vi "AprilTag Target Package Code 2.vi"() -> ()   [LabVIEW 2023]
uses:
  Camera Info.ctl
  State Machine/AprialTag Main Cluster.ctl
  State Machine/AprialTag States.ctl
  <vilib>/vision/Image Controls.llb/IMAQ Image.ctl
  Steam Type.ctl
  Camera Set Up/Event Setup Types.ctl
  <vilib>/Utility/config.llb/Read Key (String).vi
  <vilib>/Utility/config.llb/Write Key (String).vi
  <vilib>/Utility/config.llb/NI_LVConfig.lvlib
panel:
  in  "Main":enum32{"Page 1", "Page 2"}(tab)
  out "Target Pitch":dbl[](array[numeric]) caption="Tag Pitch (deg)" format="%.1f"
  out "Target Roll":dbl[](array[numeric]) caption="Tag Yaw (deg)" format="%.1f"
  out "Tag ID":dbl[](array[numeric]) caption="Tag Number"
  out "Image":T1(plugin-control)
  in  "Camera Name":string="cam0"
  in  "Settings":bool
  in  "Save":bool
  in  "Tools":bool
  out "AprilTag Fps":dbl format="%#.0f"
  out "Distance":dbl[](array[numeric]) caption="Tag Distance (in)" format="%.1f"
  out "Angle":dbl[](array[numeric]) caption="Center Angle (deg)" format="%.1f"
  in  "Home":bool
  in  "FOV":dbl=68.5
  in  "Robot Calibration Cluster":T2={"Camera Height on robot (in)"=9.5, "Camera Angle on the robot (deg)"=2.5, "Camera FOV Top to Bottom View Angle (deg)"=26.5, "Target size (in)"=6.5, "Distance to front of bumper (in)"=9.75, "Focal Length (mm)"=10.0, "Yaw Slope"=0.0} {"Focal Length (mm)" format="%#_13g"; "Distance to front of bumper (in)" format="%#_13g"; "Target size (in)" format="%#_13g"; "Camera FOV Top to Bottom View Angle (deg)" format="%#_13g"; "Camera Angle on the robot (deg)" format="%#_13g"; "Camera Height on robot (in)" format="%#_13g"}
  # "Edit the camera name to the camera that you are going to use for this target package"
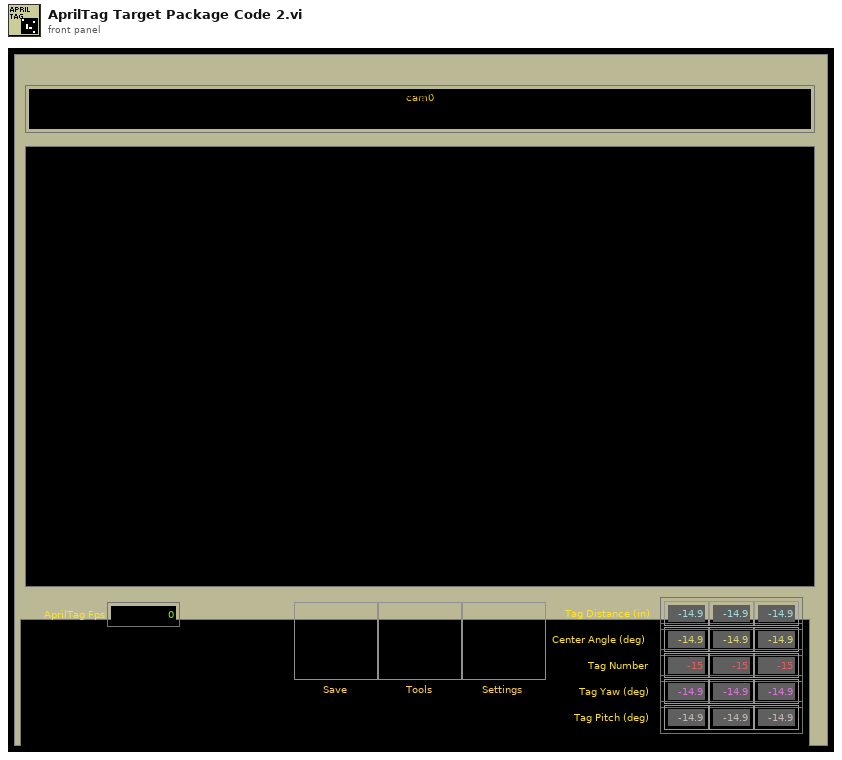
[diagram p1: front panel]
types:
  T1 = typedef "IMAQ Image.ctl" = refnum<image>
  T2 = typedef "Camera Info.ctl" = cluster{"Camera Height on robot (in)":dbl, "Camera Angle on the robot (deg)":dbl, "Camera FOV Top to Bottom View Angle (deg)":dbl, "Target size (in)":dbl, "Distance to front of bumper (in)":dbl, "Focal Length (mm)":dbl, "Yaw Slope":dbl}
  T3 = typedef "AprialTag States.ctl" = enum16{"Message Dispatcher", "INI", "Open", "Save", "Exit"}
  T4 = typedef "AprialTag Main Cluster.ctl" = cluster{"AprilTage FIFO":T3[], "Camera Name":string, "AprilTag path":path, "Control Ref's":refnum<vi>[], "Calibration Mask":T1, "Main Image":T1, "Timeout":i32, "EDIT Settings":bool, "Calibration path":path, "Camera Number":dbl}
  T5 = typedef "Steam Type.ctl" = enum8{"Unknown", "Apriltag", "Algae", "Coral"}
  T6 = typedef "Event Setup Types.ctl" = enum16{"Default", "Camera Loop Started", "Close Settings", "GreyScale", "Open Front Panel", "Save Data", "Exit"}
  T7 = cluster{"tag ID":i32, "Center":cluster{"X":dbl, "Y":dbl}, "homography matrix":dbl[], "decision margin":dbl, "Hamming Dist":i32, "corner points":cluster{"X":dbl, "Y":dbl}[], "Tag Family":string}[]
  T8 = typedef "AprilTag Target Fields.ctl" = cluster{"diameter points":cluster{"first point":cluster{"x":dbl, "y":dbl}, "projected point":cluster{"x":dbl, "y":dbl}}, "normalized center":cluster{"x":dbl, "y":dbl}, "Overall Score":dbl, "Distance (ft)":dbl, "Offset Angle":dbl, "Tag corner points":cluster{"X":dbl, "Y":dbl}[], "Tag Center":cluster{"X":dbl, "Y":dbl}, "Tag Yaw":dbl, "Tag Pitch":dbl, "AprilTag Number":i32}
  T9 = typedef "Image Type" = u32
  T10 = typedef "NI_LVConfig.lvlib/Config Data RefNum.ctl" = refnum<k1>
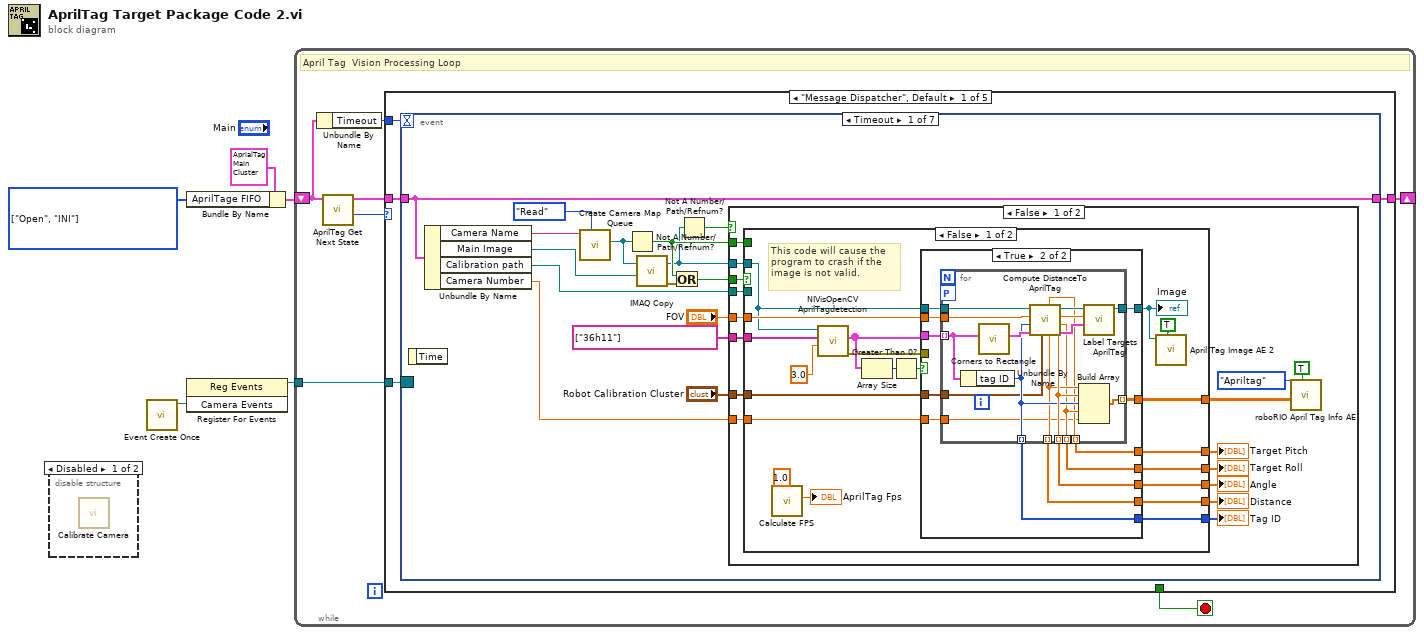
[diagram p0: block diagram]
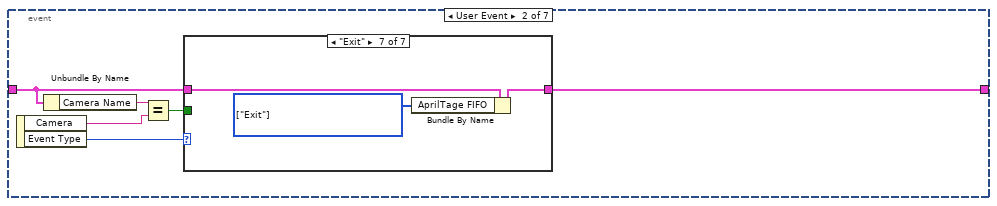
[diagram p6: hidden frame]
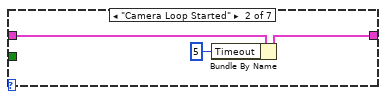
[diagram p8: hidden frame]
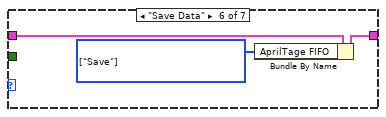
[diagram p12: hidden frame]
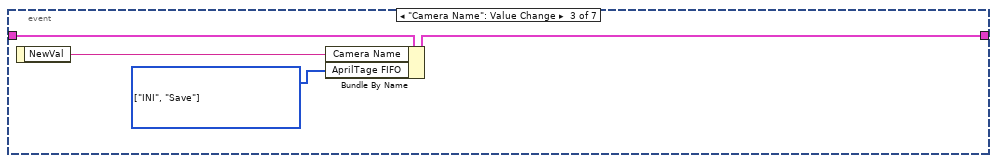
[diagram p13: hidden frame]
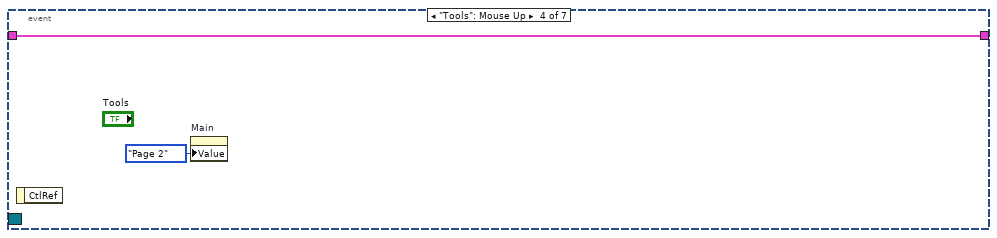
[diagram p14: hidden frame]
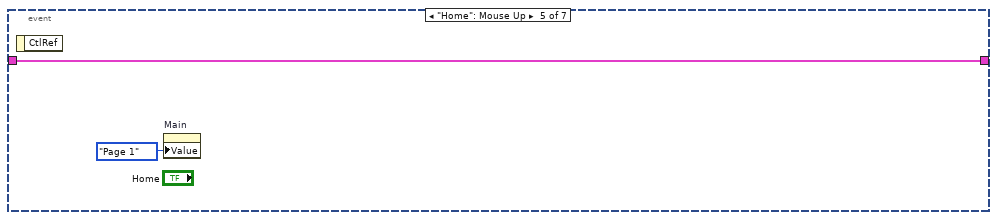
[diagram p15: hidden frame]
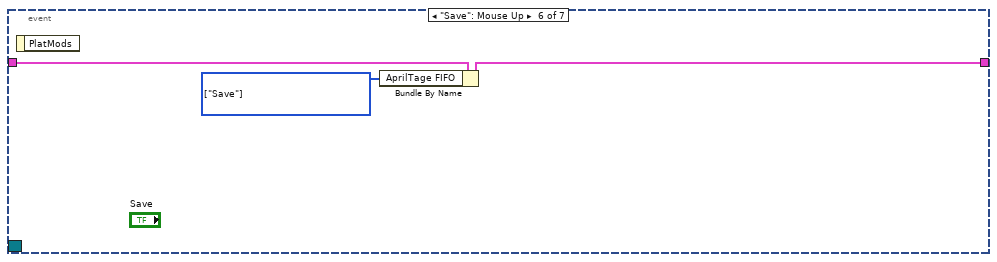
[diagram p16: hidden frame]
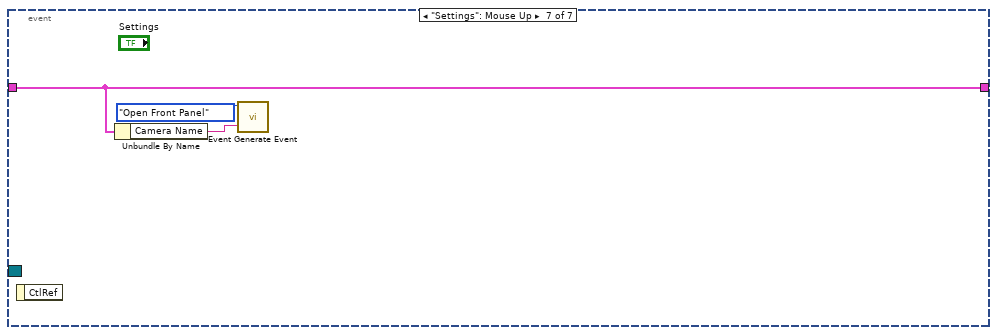
[diagram p17: hidden frame]
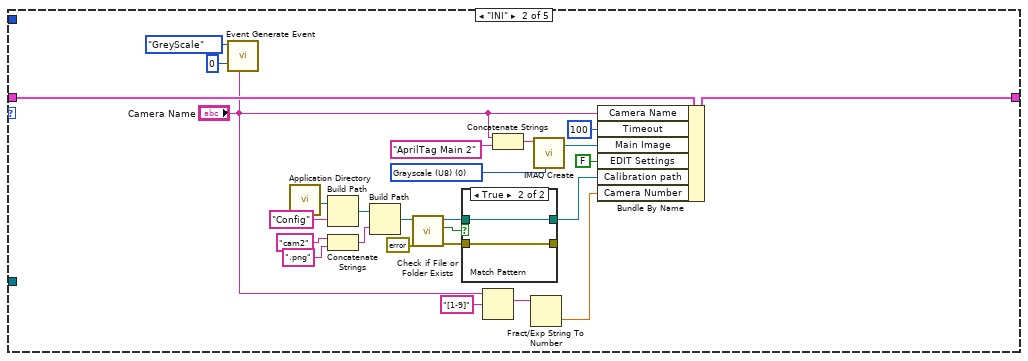
[diagram p18: hidden frame]
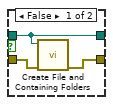
[diagram p19: hidden frame]
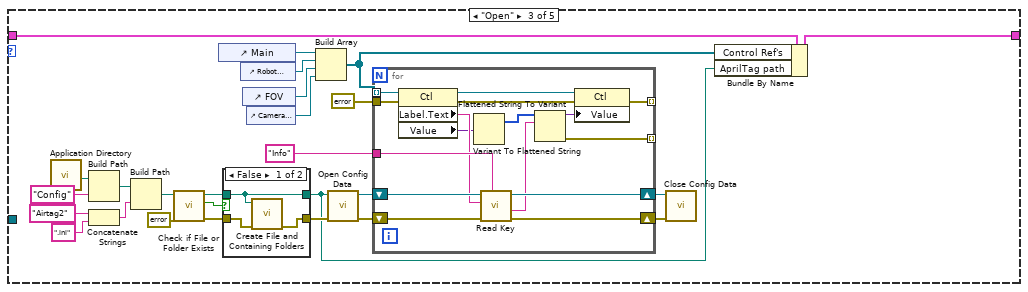
[diagram p20: hidden frame]
diagram:
  w1 = T3[] [enum."Open", enum."INI"] items=["Message Dispatcher", "INI", "Open", "Save", "Exit"] ("AprilTage FIFO")
  n1 = disable-structure shown="Disabled" {
    frame Disabled {
      n2 = call "Calibrate Camera.vi"() -> ()  [unwired: 13 in, 3 out]
    }
    frame Enabled {
    }
  }
  n3 = call "Event Create Once.vi"() -> ("Camera Events"=w5:refnum<user-event>)  [unwired: 10 in, 1 out]
  n4 = Bundle By Name(cluster=T4 {"AprilTage FIFO"=[], "Camera Name"="", "AprilTag path"=path "", "Control Ref's"=[], "Calibration Mask"=refnum, "Main Image"=refnum, "Timeout"=5, "EDIT Settings"=FALSE, "Calibration path"=path "", "Camera Number"=0.0} ("AprilTag Main Cluster out"), "AprilTage FIFO"=w1) -> (w2:T4)
  n5 = register-events(w5) -> (reference out=w4:refnum<event-registration>)  [unwired: 2 in, 1 out]
  n6 = while {
    tunnel: w4 -> [w12]
    shift-right: [w8] -> _
    shift-left: w2 -> [w6]
    stop <- w11 stop-if-true
    # "April Tag  Vision Processing Loop"
    n7 = Unbundle By Name(w6) -> ("Timeout"=w7:i32)
    n8 = call "AprilTag Get Next State.vi"("AprilTag Main Cluster in"=w6) -> ("Next State"=w9:T3, "AprilTag Main Cluster out"=w10:T4)  [unwired: 9 in]
    n9 = case shown="\"Message Dispatcher\", Default" w9 {
      tunnel: w12 -> [w16 _ _ _ _]
      tunnel: [_ _ _ _ TRUE] -> w11
      tunnel: w10 -> [w14 w154 w171 w210 w227]
      tunnel: [w15 w153 w169 w210 w227] -> w8
      tunnel: w7 -> [w13 _ _ _ _]
      frame "Message Dispatcher", Default {
        n10 = event shown="[0] Timeout" {
          selector: w16 -> [_ _ _ _ _ _ _]
          dyn-events: _ -> [_ _ _ _ _ _ _]
          timeout: w13 -> [_ _ _ _ _ _ _]
          tunnel: w14 -> [w31 w99 w118 w119 w121 w125 w127]
          tunnel: [w31 w101 w117 w119 w121 w124 w127] -> w15
          event Timeout {
            n11 = event-data() -> ()  [unwired: 1 in, 1 out]
            n12 = Unbundle By Name(w31) -> ("Camera Name"=w24:string, "Main Image"=w20:T1, "Calibration path"=w30:path, "Camera Number"=w17:dbl)
            n13 = call "Create Camera Map Queue.vi"("Action"=enum16{"Read", "Write"}."Read", "Camera"=w24) -> ("Image out"=w23:T1)  [unwired: 8 in, 1 out]
            n14 = Not A Number/Path/Refnum?(number/path/refnum=w23) -> (NaN/Path/Refnum?=w26:bool)
            n15 = call "IMAQ Copy"("Image Dst"=w20, "Image Src"=w23) -> ("error out"=w21:errorcluster, "Image Dst Out"=w19:T1)  [unwired: 4 in]
            n16 = Or(x=w26, y=w21) -> (x .or. y?=w22:bool)
            n17 = Not A Number/Path/Refnum?(number/path/refnum=w19) -> (NaN/Path/Refnum?=w18:bool)
            n18 = case shown="False" w18 {
              tunnel: w30 -> [w44 _]
              tunnel: string[] ["36h11"] ("Tag Familys") -> [w43 _]
              tunnel: "FOV" -> [w42 _]
              tunnel: "Robot Calibration Cluster" -> [w41 _]
              tunnel: w26 -> [w40 _]
              tunnel: w22 -> [w34 _]
              tunnel: w19 -> [w33 _]
              tunnel: w17 -> [w32 _]
              frame False {
                n19 = case shown="False" w34 {
                  tunnel: w43 -> [w67 _]
                  tunnel: w42 -> [w66 _]
                  tunnel: w41 -> [w65 _]
                  tunnel: [w56 _] -> w46
                  tunnel: w40 -> [_ _]
                  tunnel: w44 -> [_ _]
                  tunnel: [w55 _] -> w39
                  tunnel: [w54 _] -> w38
                  tunnel: [w53 _] -> w37
                  tunnel: [w52 _] -> w36
                  tunnel: [w51 _] -> w35
                  tunnel: w33 -> [w49 _]
                  tunnel: w32 -> [w48 _]
                  frame False {
                    # "This code will cause the program to crash if the image is not valid."
                    n20 = call "Calculate FPS.vi"("Frames Processed"=1.0) -> ("Fps"=→"AprilTag Fps":dbl)  [unwired: 10 in]
                    n21 = call "NIVisOpenCV AprilTagdetection.vi"("decimate"=3.0, "Tag Familys"=w67, "Image Src"=w49) -> ("error out"=w61:errorcluster, "Detected Tags"=w64:T7)  [unwired: 5 in, 2 out]
                    n22 = Array Size(array=w64) -> (size(s)=w63:i32)
                    n23 = Greater Than 0?(x=w63) -> (x > 0?=w62:bool)
                    n24 = case shown="True" w62 {
                      tunnel: w49 -> [w68 w80]
                      tunnel: w64 -> [_ w79]
                      tunnel: [w68 w78] -> w60
                      tunnel: w61 -> [_ _]
                      tunnel: w66 -> [_ w77]
                      tunnel: w65 -> [_ w76]
                      tunnel: [_ w75] -> w56
                      tunnel: [_ w74] -> w55
                      tunnel: [_ w73] -> w54
                      tunnel: [_ w72] -> w53
                      tunnel: [_ w71] -> w52
                      tunnel: [_ w70] -> w51
                      tunnel: w48 -> [_ w69]
                      frame False {
                      }
                      frame True {
                        n25 = for {
                          tunnel: w79 -> [w93] mode=indexing
                          tunnel: w80 -> [w94]
                          tunnel: [w95] -> w78
                          tunnel: [w87] -> w72 mode=indexing
                          tunnel: [w85] -> w70 mode=indexing
                          tunnel: [w89] -> w71 mode=indexing
                          tunnel: w77 -> [w88]
                          tunnel: w76 -> [w86]
                          tunnel: [w84] -> w73 mode=indexing
                          tunnel: [w83] -> w75 mode=indexing
                          tunnel: [w82] -> w74 mode=indexing
                          workers-P: _ -> [_]
                          tunnel: w69 -> [w81]
                          n26 = Unbundle By Name(w93) -> ("tag ID"=w87:i32)
                          n27 = call "Corners to Rectangle.vi"("tag info"=w93) -> ("output cluster"=w92:T8)  [unwired: 10 in]
                          n28 = call "Compute DistanceTo AprilTag.vi"("Robot Calibration Cluster"=w86, "results"=w92, "AprilTag Number"=w87, "FOV Left to Right (deg)"=w88, "Image Src"=w94) -> ("results out"=w91:T8, "Target Yaw (deg)"=w84:dbl, "Offset Angle"=w89:dbl, "Image Dst Out"=w90:T1, "Distance from target (in)"=w85:dbl, "Target Pitch (deg)"=w82:dbl)  [unwired: 1 in]
                          n29 = Build Array(w85, w89, w87, w84, w81) -> (w83:dbl[])
                          n30 = call "Label Targets AprilTagl.vi"("results"=w91, "Angle"=w89, "Image in"=w90) -> ("Image out"=w95:T1)  [unwired: 8 in]
                        }
                      }
                    }
                    "Image" <- w60
                    n31 = call "April Tag Image AE 2.vi"("Update"=TRUE, "Ball Image in"=w60) -> ()  [unwired: 9 in, 1 out]
                  }
                  frame True {
                  }
                }
                "Distance" <- w35
                "Angle" <- w36
                "Tag ID" <- w37
                "Target Roll" <- w38
                "Target Pitch" <- w39
                n32 = call "roboRIO April Tag Info AE.vi"("Update"=TRUE, "Info in"=w46, "Stream Type"=Steam_Type."Apriltag") -> ()  [unwired: 8 in, 1 out]
              }
              frame True {
              }
            }
          }
          event User Event {
            n33 = event-data() -> ("Camera"=w97:string, "Event Type"=w100:T6)  [unwired: 1 in]
            n34 = Unbundle By Name(w99) -> ("Camera Name"=w98:string)
            n35 = Equal?(x=w98, y=w97) -> (x = y?=w96:bool)
            n36 = case shown="\"Exit\"" w100 {
              tunnel: w99 -> [w102 w105 w106 w107 w108 w111 w114]
              tunnel: [w102 w104 w106 w107 w108 w110 w113] -> w101
              tunnel: w96 -> [_ _ _ _ _ _ _]
              frame "Default" {
              }
              frame "Camera Loop Started" {
                n37 = Bundle By Name(cluster=w105, "Timeout"=5) -> (w104:T4)
              }
              frame "Close Settings" {
              }
              frame "GreyScale" {
              }
              frame "Open Front Panel" {
              }
              frame "Save Data" {
                w109 = T3[] [enum."Save"] items=["Message Dispatcher", "INI", "Open", "Save", "Exit"] ("AprilTage FIFO")
                n38 = Bundle By Name(cluster=w111, "AprilTage FIFO"=w109) -> (w110:T4)
              }
              frame "Exit" {
                w112 = T3[] [enum."Exit"] items=["Message Dispatcher", "INI", "Open", "Save", "Exit"] ("AprilTage FIFO")
                n39 = Bundle By Name(cluster=w114, "AprilTage FIFO"=w112) -> (w113:T4)
              }
            }
          }
          event "Camera Name": Value Change {
            w116 = T3[] [enum."INI", enum."Save"] items=["Message Dispatcher", "INI", "Open", "Save", "Exit"] ("AprilTage FIFO")
            n40 = event-data() -> ("NewVal"=w115:string)  [unwired: 1 in]
            n41 = Bundle By Name(cluster=w118, "Camera Name"=w115, "AprilTage FIFO"=w116) -> (w117:T4)
          }
          event "Tools": Mouse Up {
            n42 = event-data() -> ()  [unwired: 1 in, 1 out]
            n43 = property on="Main" class="TabCtl (strict)"("Value"=enum32{"Page 1", "Page 2"}."Page 2" ("Main")) -> ()  [unwired: 2 in, 2 out]
          }
          event "Home": Mouse Up {
            n44 = event-data() -> ()  [unwired: 1 in, 1 out]
            n45 = property on="Main" class="TabCtl (strict)"("Value"=enum32{"Page 1", "Page 2"}."Page 1" ("Main")) -> ()  [unwired: 2 in, 2 out]
          }
          event "Save": Mouse Up {
            w123 = T3[] [enum."Save"] items=["Message Dispatcher", "INI", "Open", "Save", "Exit"] ("AprilTage FIFO")
            n46 = event-data() -> ()  [unwired: 1 in, 1 out]
            n47 = Bundle By Name(cluster=w125, "AprilTage FIFO"=w123) -> (w124:T4)
          }
          event "Settings": Mouse Up {
            n48 = event-data() -> ()  [unwired: 1 in, 1 out]
            n49 = Unbundle By Name(w127) -> ("Camera Name"=w126:string)
            n50 = call "Event Generate Event.vi"("Camera Name"=w126, "Event Type"=Event_Setup_Types."Open Front Panel") -> ()  [unwired: 10 in]
          }
        }
      }
      frame "INI" {
        w151 = T9 0 items=["Grayscale (U8)", "Grayscale (I16)", "Grayscale (SGL)", "Complex (CSG)", "RGB (U32)", "HSL (U32)", "RGB (U64)", "Grayscale (U16)"] ("Image Type")
        n51 = call "Event Generate Event.vi"("Camera Name"="Camera Name", "Setpoint"=i64 0, "Event Type"=Event_Setup_Types."GreyScale") -> ()  [unwired: 9 in]
        n52 = call <vilib>:"Application Directory.vi"() -> ("Application Directory"=w144:path)
        n53 = Build Path(base path=w144, name or relative path="Config") -> (appended path=w142:path)
        n54 = Concatenate Strings("cam2" ("string"), ".png" ("name or relative path")) -> (w146:string)
        n55 = Build Path(base path=w142, name or relative path=w146) -> (appended path=w141:path)
        n56 = call <vilib>:"Check if File or Folder Exists.vi"("error in (no error)"=errorcluster {"status"=FALSE, "code"=0, "source"=""}, "path"=w141) -> ("error out"=w138:errorcluster, "file or folder exists?"=w139:bool, "dup path"=w140:path)  [unwired: 7 in]
        n57 = case shown="True" w139 {
          tunnel: [w157 w158] -> _
          tunnel: w140 -> [w156 w159]
          tunnel: [w156 w159] -> w135
          tunnel: w138 -> [w155 w158]
          frame False {
            n58 = call <vilib>:"Create File and Containing Folders.vi"("error in (no error)"=w155, "file path"=w156) -> ("error out"=w157:errorcluster)  [unwired: 8 in, 1 out]
          }
          frame True {
          }
        }
        n59 = Match Pattern(string="Camera Name", regular expression="[1-9]") -> (match substring=w131:string)  [unwired: 1 in, 3 out]
        n60 = Concatenate Strings("Camera Name", "AprilTag Main 2" ("string")) -> (w150:string)
        n61 = Fract/Exp String To Number(string=w131) -> (number=w129:dbl)  [unwired: 3 in, 1 out]
        n62 = call "IMAQ Create"("Image Name"=w150, "Image Type"=w151) -> ("New Image"=w148:T1)  [unwired: 2 in, 2 out]
        n63 = Bundle By Name(cluster=w154, "Camera Name"="Camera Name", "Timeout"=100, "Main Image"=w148, "EDIT Settings"=FALSE, "Calibration path"=w135, "Camera Number"=w129) -> (w153:T4)
      }
      frame "Open" {
        n64 = call <vilib>:"Application Directory.vi"() -> ("Application Directory"=w174:path)
        n65 = Build Path(base path=w174, name or relative path="Config") -> (appended path=w172:path)
        n66 = Concatenate Strings("Airtag2" ("string"), ".ini" ("name or relative path")) -> (w185:string)
        n67 = Build Path(base path=w172, name or relative path=w185) -> (appended path=w165:path)
        n68 = call <vilib>:"Check if File or Folder Exists.vi"("error in (no error)"=errorcluster {"status"=FALSE, "code"=0, "source"=""}, "path"=w165) -> ("error out"=w161:errorcluster, "file or folder exists?"=w163:bool, "dup path"=w164:path)  [unwired: 7 in]
        n69 = control-ref of="Main"() -> (w180:refnum<vi>)
        n70 = case shown="False" w163 {
          tunnel: [w188 w189] -> w175
          tunnel: w164 -> [w187 w190]
          tunnel: [w187 w190] -> w162
          tunnel: w161 -> [w186 w189]
          frame False {
            n71 = call <vilib>:"Create File and Containing Folders.vi"("error in (no error)"=w186, "file path"=w187) -> ("error out"=w188:errorcluster)  [unwired: 8 in, 1 out]
          }
          frame True {
          }
        }
        n72 = control-ref of="Robot Calibration Cluster"() -> (w179:refnum<vi>)
        n73 = control-ref of="FOV"() -> (w178:refnum<vi>)
        n74 = control-ref of="Camera Name"() -> (w170:refnum<vi>)
        n75 = Build Array(w180, w179, w178, w170) -> (w168:refnum<vi>[])
        n76 = call <vilib>:"Open Config Data.vi"("error in (no error)"=w175, "configuration file path"=w162) -> ("error out"=w181:errorcluster, "refnum"=w184:T10)  [unwired: 7 in, 1 out]
        n77 = for {
          tunnel: "Info" ("Camera Name") -> [w203]
          tunnel: w168 -> [w201] mode=indexing
          shift-right: [w205] -> w183
          shift-left: w184 -> [w206]
          shift-right: [w204] -> w182
          shift-left: w181 -> [w202]
          tunnel: [w196] -> _ mode=indexing
          tunnel: errorcluster {"status"=FALSE, "code"=0, "source"=""} ("error out") -> [w195]
          tunnel: [w191] -> _ mode=indexing
          n78 = property class="Ctl"(reference=w201, error in=w195) -> (reference out=w199:refnum<vi>, error out=w197:errorcluster, "Label.Text"=w200:string, "Value"=w193:variant)
          n79 = Variant To Flattened String(Variant=w193) -> (1:w192:i16[])  [unwired: 1 out]
          n80 = call-poly <vilib>:"Read Key.vi"("section"=w203, "error in (no error)"=w202, "key"=w200, "refnum"=w206) -> ("error out"=w204:errorcluster, "value"=w198:string, "refnum out"=w205:T10)  [unwired: 4 in, 1 out]
          n81 = Flattened String To Variant(6:w198, 7:w192) -> (0:w191:errorcluster, 3:w194:variant)  [unwired: 1 in]
          n82 = property class="Ctl"(reference=w199, error in=w197, "Value"=w194) -> (error out=w196:errorcluster)  [unwired: 1 out]
        }
        n83 = call <vilib>:"Close Config Data.vi"("error in (no error)"=w182, "refnum"=w183) -> ()  [unwired: 8 in, 2 out]
        n84 = Bundle By Name(cluster=w171, "Control Ref's"=w168, "AprilTag path"=w162) -> (w169:T4)
      }
      frame "Save" {
        n85 = Unbundle By Name(w210) -> ("Control Ref's"=w208:refnum<vi>[], "AprilTag path"=w209:path)
        n86 = call <vilib>:"Open Config Data.vi"("configuration file path"=w209) -> ("error out"=w211:errorcluster, "refnum"=w214:T10)  [unwired: 8 in, 1 out]
        n87 = for {
          tunnel: "Info" ("Camera Name") -> [w220]
          shift-right: [w223] -> w213
          shift-left: w214 -> [w224]
          shift-right: [w222] -> w212
          shift-left: w211 -> [w221]
          tunnel: w208 -> [w215] mode=indexing
          n88 = property class="Ctl"(reference=w215, error in=w221) -> (error out=w217:errorcluster, "Label.Text"=w219:string, "Value"=w218:variant)  [unwired: 1 out]
          n89 = Variant To Flattened String(Variant=w218) -> (data string=w216:string)  [unwired: 1 out]
          n90 = call-poly <vilib>:"Write Key.vi"("section"=w220, "error in (no error)"=w217, "value"=w216, "key"=w219, "refnum"=w224) -> ("error out"=w222:errorcluster, "refnum out"=w223:T10)  [unwired: 4 in, 1 out]
        }
        n91 = call <vilib>:"Close Config Data.vi"("error in (no error)"=w212, "refnum"=w213) -> ()  [unwired: 8 in, 2 out]
      }
      frame "Exit" {
        n92 = Unbundle By Name(w227) -> ("Calibration Mask"=w226:T1, "Main Image"=w225:T1)
        n93 = call "IMAQ Dispose"("Image"=w226) -> ()  [unwired: 5 in, 1 out]
        n94 = call "IMAQ Dispose"("Image"=w225) -> ()  [unwired: 5 in, 1 out]
      }
    }
  }
